vi "Producer Consumer.vi"() -> ()   [LabVIEW 2020]
panel:
  out "Error Out":errorcluster
  in  "Error In":errorcluster
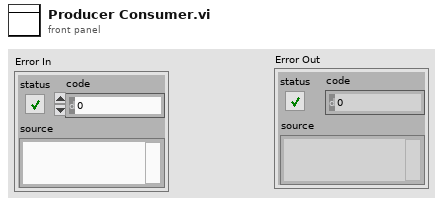
[diagram p1: front panel]
types:
  T1 = enum16{"Create", "Enqueue", "Dequeue", "Enstack", "Flush", "Destroy"}
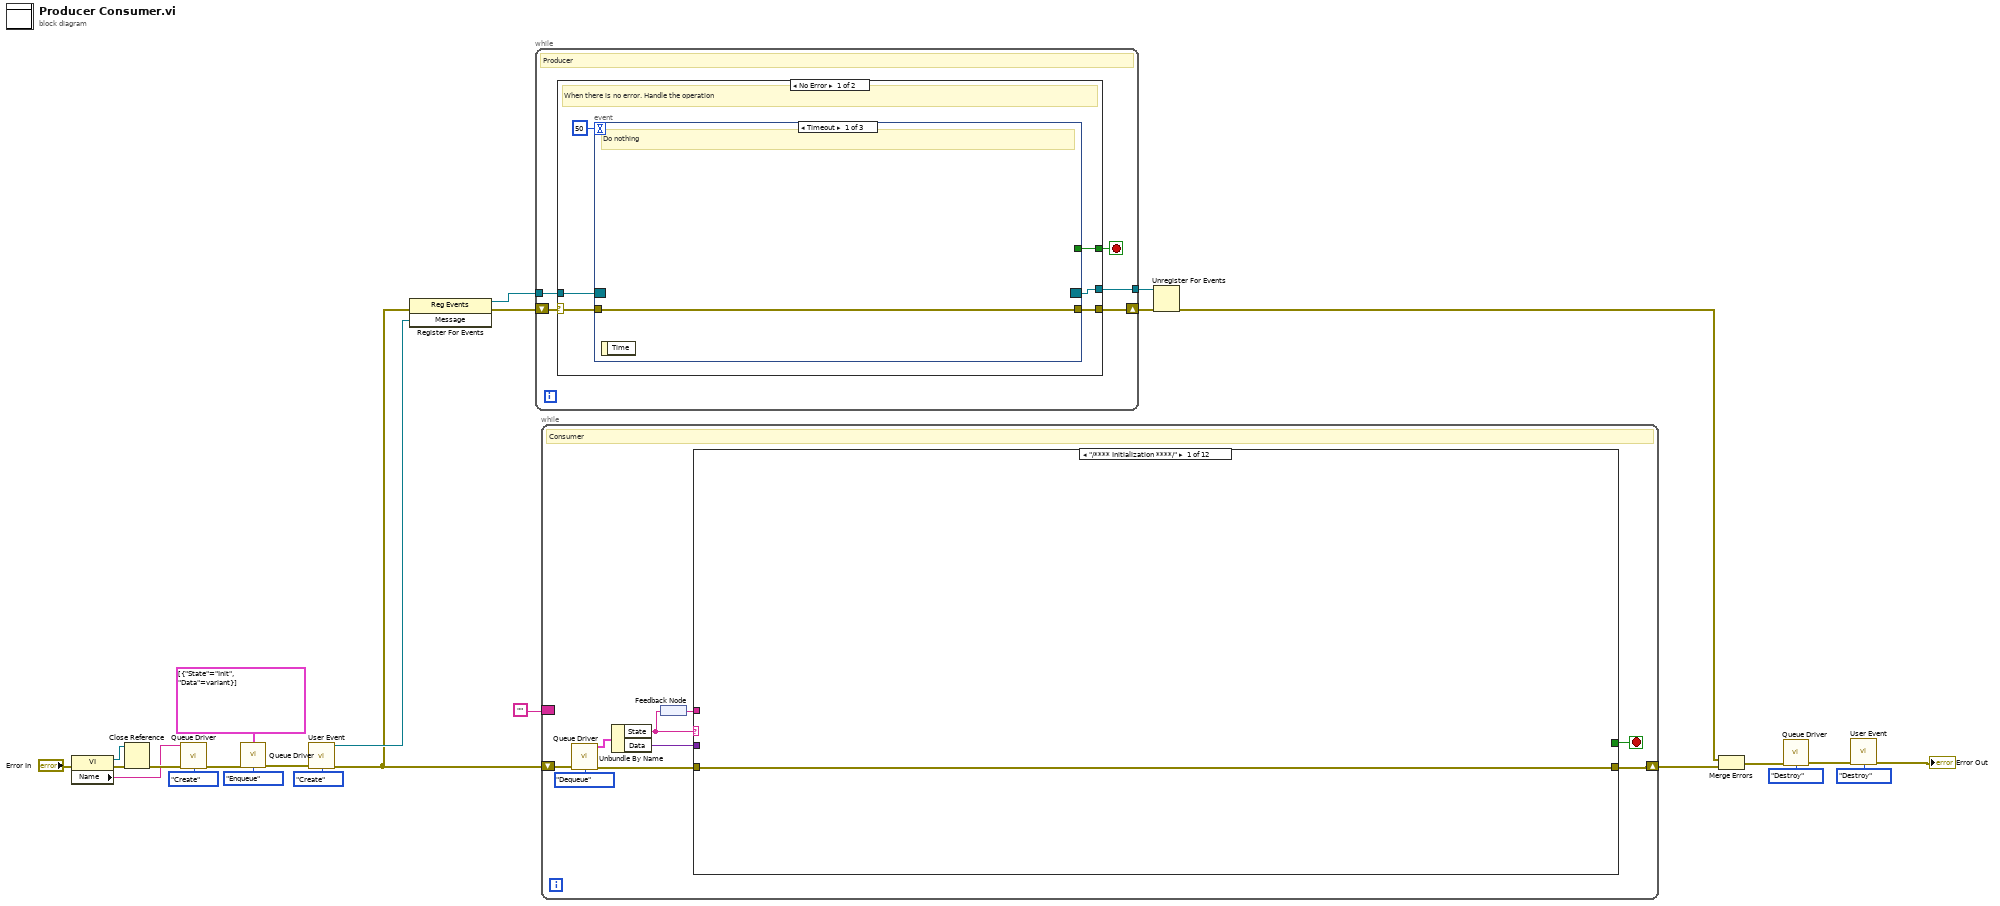
[diagram p0: block diagram]
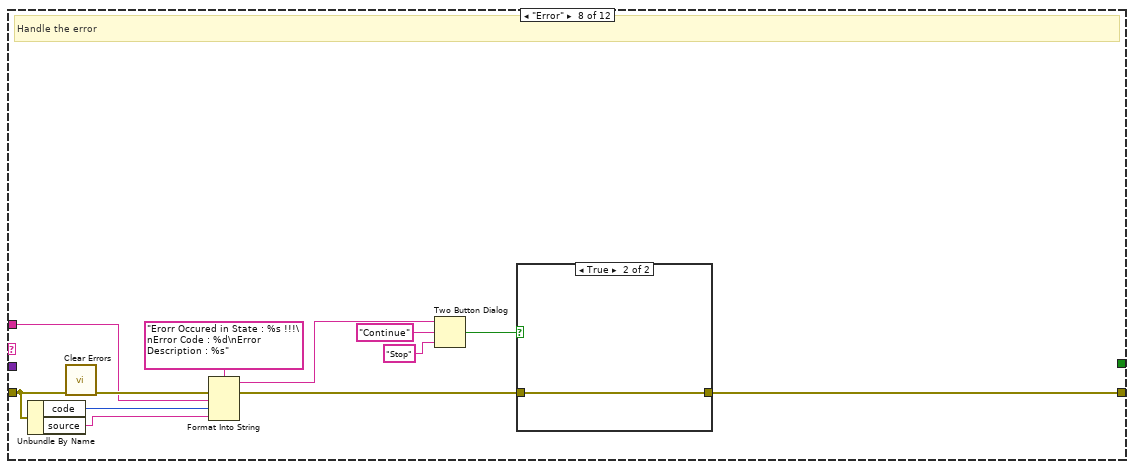
[diagram p8: hidden frame]
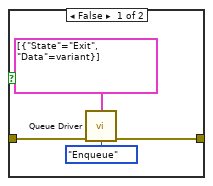
[diagram p9: hidden frame]
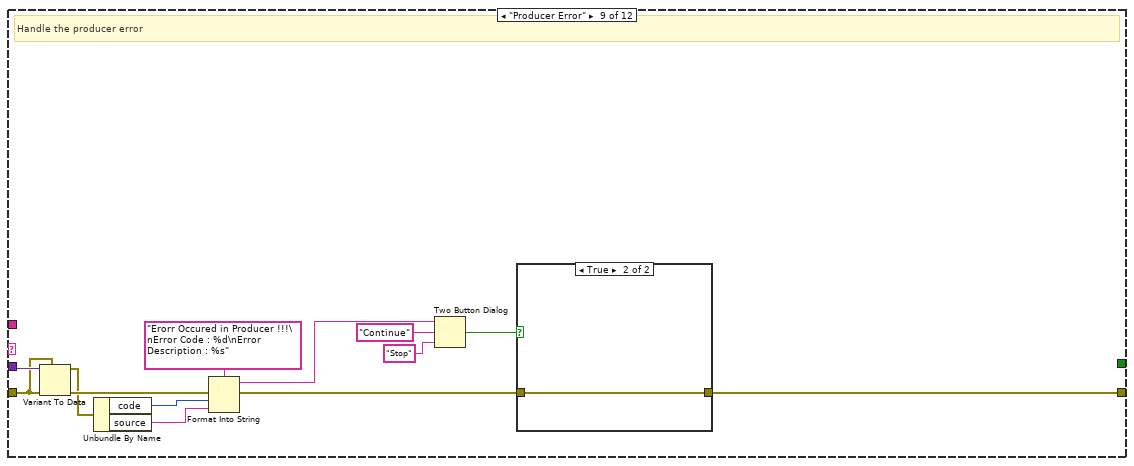
[diagram p10: hidden frame]
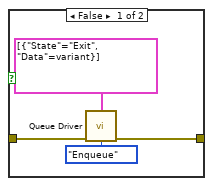
[diagram p11: hidden frame]
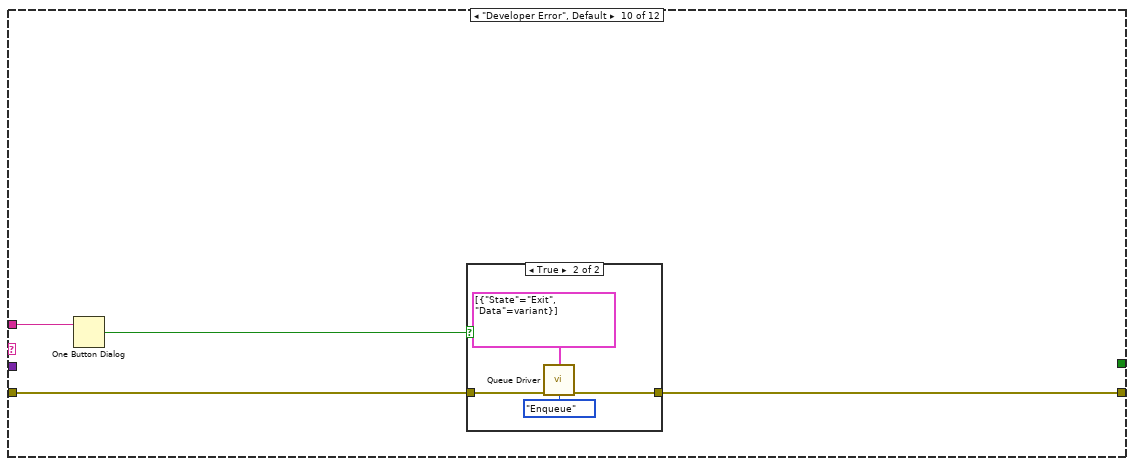
[diagram p12: hidden frame]
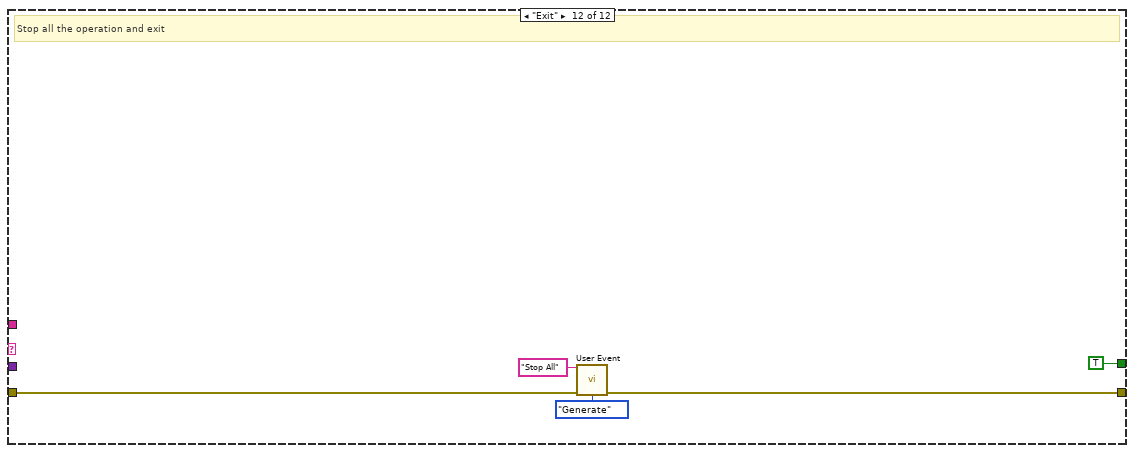
[diagram p15: hidden frame]
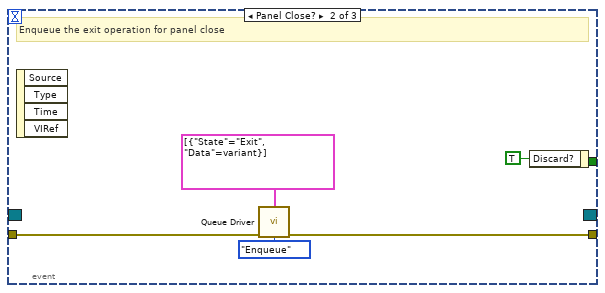
[diagram p16: hidden frame]
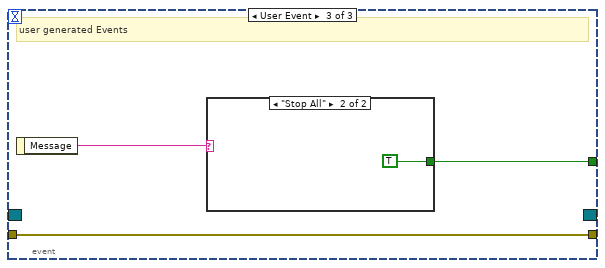
[diagram p17: hidden frame]
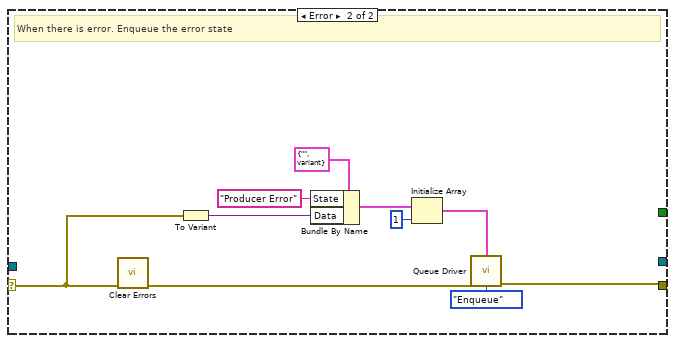
[diagram p19: hidden frame]
diagram:
  n1 = property class="VI"(error in="Error In") -> (reference out=w18:refnum<vi>, error out=w20:errorcluster, "Name"=w17:string)  [unwired: 1 in]
  n2 = Close Reference(reference=w18, error in (no error)=w20) -> (error out=w19:errorcluster)
  n3 = call "Queue Driver.vi"("Queue Name"=w17, "Error In"=w19, "Q Operations"=T1."Create") -> ("Error Out"=w16:errorcluster)  [unwired: 11 in, 1 out]
  n4 = call "Queue Driver.vi"("State[]"=cluster{"State":string, "Data":variant}[] [{"State"="Init", "Data"=variant}], "Error In"=w16, "Q Operations"=T1."Enqueue") -> ("Error Out"=w15:errorcluster)  [unwired: 11 in, 1 out]
  n5 = call "User Event.vi"("Error In"=w15, "Enum"=enum16{"Create", "Generate", "Destroy"}."Create") -> ("Message"=w11:refnum<user-event>, "Error Out"=w10:errorcluster)  [unwired: 12 in]
  n6 = register-events(error in=w10, w11) -> (reference out=w9:refnum<event-registration>, error out=w12:errorcluster)  [unwired: 1 in]
  n7 = while {
    shift-right: [w29] -> w24
    shift-left: w12 -> [w30]
    tunnel: w9 -> [w28]
    tunnel: [w27] -> w7
    stop <- w26 stop-if-true
    # "Producer"
    n8 = case shown="No Error" w30 {
      selector: w30 -> [w36 w50]
      tunnel: [w35 w53] -> w29
      tunnel: w28 -> [w33 _]
      tunnel: [w32 _] -> w27
      tunnel: [w31 _] -> w26
      frame No Error {
        # "When there is no error. Handle the operation"
        n9 = event shown="[0] Timeout" {
          selector: w33 -> [_ _ _]
          dyn-events: [_ _ _] -> w32
          timeout: 50 -> [_ _ _]
          tunnel: [w37 w39 w44] -> w35
          tunnel: w36 -> [w37 w39 w44]
          tunnel: [_ _ w42] -> w31
          event Timeout {
            # "Do nothing"
            n10 = event-data() -> ()  [unwired: 1 in, 1 out]
          }
          event Panel Close? {
            # "Enqueue the exit operation for panel close"
            n11 = event-data() -> ()  [unwired: 1 in, 4 out]
            n12 = call "Queue Driver.vi"("State[]"=cluster{"State":string, "Data":variant}[] [{"State"="Exit", "Data"=variant}], "Error In"=w39, "Q Operations"=T1."Enqueue") -> ()  [unwired: 11 in, 2 out]
            n13 = event-data("Discard?"=TRUE) -> ()  [unwired: 1 in, 1 out]
          }
          event User Event {
            # "user generated Events"
            n14 = event-data() -> ("Message"=w43:string)  [unwired: 1 in]
            n15 = case shown="\"Stop All\"" w43 {
              tunnel: [_ TRUE] -> w42
              frame Default {
              }
              frame "Stop All" {
              }
            }
          }
        }
      }
      frame Error {
        # "When there is error. Enqueue the error state"
        n16 = call <vilib>:"Clear Errors.vi"("error in (no error)"=w50) -> ("error out"=w54:errorcluster)  [unwired: 5 in, 1 out]
        n17 = To Variant(anything=w50) -> (Variant=w49:variant)
        n18 = Bundle By Name(cluster=cluster{"State":string, "Data":variant} {"State"="", "Data"=variant} ("Dequeued State"), "State"="Producer Error", "Data"=w49) -> (w48:cluster{"State":string, "Data":variant})
        n19 = Initialize Array(w48, 1 ("dimension size")) -> (w47:cluster{"State":string, "Data":variant}[])
        n20 = call "Queue Driver.vi"("State[]"=w47, "Error In"=w54, "Q Operations"=T1."Enqueue") -> ("Error Out"=w53:errorcluster)  [unwired: 11 in, 1 out]
      }
    }
  }
  n21 = while {
    shift-right: [w60] -> w25
    shift-left: w10 -> [w63]
    border: "" -> [_]
    stop <- w58 stop-if-true
    # "Consumer"
    n22 = call "Queue Driver.vi"("Error In"=w63, "Q Operations"=T1."Dequeue") -> ("Dequeued State"=w62:cluster{"State":string, "Data":variant}, "Error Out"=w61:errorcluster)  [unwired: 12 in]
    n23 = Unbundle By Name(w62) -> ("State"=w57:string, "Data"=w59:variant)
    n24 = feedback-in #1(w57) -> ()
    n25 = feedback #1() -> (w56:string)
    n26 = case shown="\"/**** Initialization ****/\"" w57 {
      tunnel: w61 -> [w65 w66 w67 w68 w69 w70 w71 w82 w90 w109 w116 w119]
      tunnel: [w65 w66 w67 w68 w69 w70 w71 w73 w94 w108 w116 w118] -> w60
      tunnel: w59 -> [_ _ _ _ _ _ _ _ w91 _ _ _]
      tunnel: [_ _ _ _ _ _ _ _ _ _ _ TRUE] -> w58
      tunnel: w56 -> [_ _ _ _ _ _ _ w78 _ w110 _ _]
      frame "/**** Initialization ****/" {
      }
      frame "Init" {
        # "Initialize the values in the data cluster"
      }
      frame "/**** FP Related *****/" {
      }
      frame "FP Update" {
        # "Update the front panel controls"
      }
      frame "/***** functionalities ****/" {
      }
      frame "" {
        # "Do nothing"
      }
      frame "/***** Error States ****/" {
      }
      frame "Error" {
        # "Handle the error"
        n27 = Unbundle By Name(w82) -> ("code"=w80:i32, "source"=w79:string)
        n28 = call <vilib>:"Clear Errors.vi"("error in (no error)"=w82) -> ("error out"=w83:errorcluster)  [unwired: 5 in, 1 out]
        n29 = Format Into String(format string="Erorr Occured in State : %s !!!\nError Code : %d\nError Description : %s", error in=w83, w78, w80, w79) -> (resulting string=w77:string, error out=w74:errorcluster)  [unwired: 1 in]
        n30 = Two Button Dialog(message=w77, 1:"Stop" ("F button name (\"Cancel\")"), 2:"Continue" ("T button name (\"OK\")")) -> (T button?=w72:bool)
        n31 = case shown="True" w72 {
          tunnel: w74 -> [w86 w88]
          tunnel: [w85 w88] -> w73
          frame False {
            n32 = call "Queue Driver.vi"("State[]"=cluster{"State":string, "Data":variant}[] [{"State"="Exit", "Data"=variant}], "Error In"=w86, "Q Operations"=T1."Enqueue") -> ("Error Out"=w85:errorcluster)  [unwired: 11 in, 1 out]
          }
          frame True {
          }
        }
      }
      frame "Producer Error" {
        # "Handle the producer error"
        n33 = Variant To Data(error in=w90, type=w90, Variant=w91) -> (data=w89:errorcluster, error out=w92:errorcluster)
        n34 = Unbundle By Name(w89) -> ("code"=w100:i32, "source"=w99:string)
        n35 = Format Into String(format string="Erorr Occured in Producer !!!\nError Code : %d\nError Description : %s", error in=w92, w100, w99) -> (resulting string=w98:string, error out=w95:errorcluster)  [unwired: 1 in]
        n36 = Two Button Dialog(message=w98, 1:"Stop" ("F button name (\"Cancel\")"), 2:"Continue" ("T button name (\"OK\")")) -> (T button?=w93:bool)
        n37 = case shown="True" w93 {
          tunnel: w95 -> [w104 w106]
          tunnel: [w103 w106] -> w94
          frame False {
            n38 = call "Queue Driver.vi"("State[]"=cluster{"State":string, "Data":variant}[] [{"State"="Exit", "Data"=variant}], "Error In"=w104, "Q Operations"=T1."Enqueue") -> ("Error Out"=w103:errorcluster)  [unwired: 11 in, 1 out]
          }
          frame True {
          }
        }
      }
      frame "Developer Error", Default {
        n39 = One Button Dialog(message=w110) -> (true=w107:bool)  [unwired: 1 in]
        n40 = case shown="True" w107 {
          tunnel: w109 -> [w111 w114]
          tunnel: [w111 w113] -> w108
          frame False {
          }
          frame True {
            n41 = call "Queue Driver.vi"("State[]"=cluster{"State":string, "Data":variant}[] [{"State"="Exit", "Data"=variant}], "Error In"=w114, "Q Operations"=T1."Enqueue") -> ("Error Out"=w113:errorcluster)  [unwired: 11 in, 1 out]
          }
        }
      }
      frame "/***** Exit States ****/" {
      }
      frame "Exit" {
        # "Stop all the operation and exit"
        n42 = call "User Event.vi"("Event Data"="Stop All", "Error In"=w119, "Enum"=enum16{"Create", "Generate", "Destroy"}."Generate") -> ("Error Out"=w118:errorcluster)  [unwired: 11 in, 1 out]
      }
    }
  }
  n43 = Unregister For Events(event registration refnum=w7, error in=w24) -> (error out=w8:errorcluster)
  n44 = Merge Errors(w8, w25) -> (w4:errorcluster)
  n45 = call "Queue Driver.vi"("Error In"=w4, "Q Operations"=T1."Destroy") -> ("Error Out"=w2:errorcluster)  [unwired: 12 in, 1 out]
  n46 = call "User Event.vi"("Error In"=w2, "Enum"=enum16{"Create", "Generate", "Destroy"}."Destroy") -> ("Error Out"=→"Error Out":errorcluster)  [unwired: 12 in, 1 out]
